vi "Send_Demand_controlword.vi"(0 "UDP connection ID out":refnum<k16>, 1 "Inner TRACK":T1={"Position"=100.0, "Rate"=100.0, "Acceleration"=100.0}, 2 "Middle TRACK":T1={"Position"=100.0, "Rate"=100.0, "Acceleration"=100.0}, 3 "Outer TRACK":T1={"Position"=100.0, "Rate"=100.0, "Acceleration"=100.0}, 5 "IP address in":u32=44, 12 "error in":errorcluster, 13 "ReadOnly":bool) -> (4 "UDP connection ID out":refnum<k16>, 6 "IP address out":u32=44, 8 "concatenated string":string, 14 "error out":errorcluster)   [LabVIEW 2017]
panel:
  in  "Inner P":cluster{dbl}
  in  "Middle P":cluster{dbl}
  in  "Outer P":cluster{dbl}
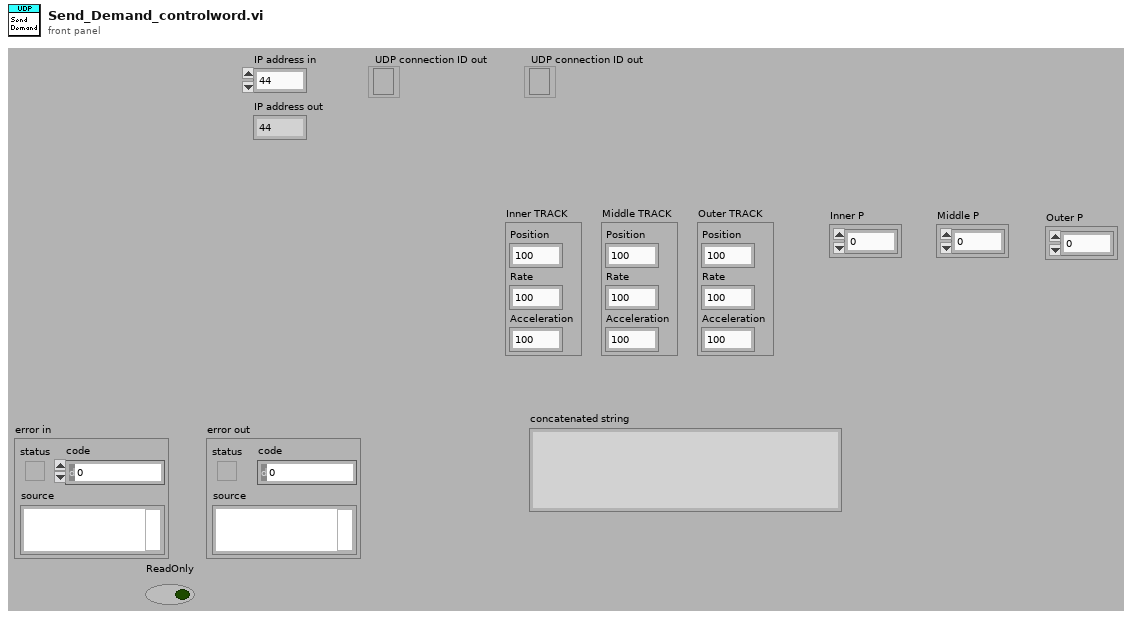
[diagram p1: front panel]
types:
  T1 = cluster{"Position":dbl, "Rate":dbl, "Acceleration":dbl}
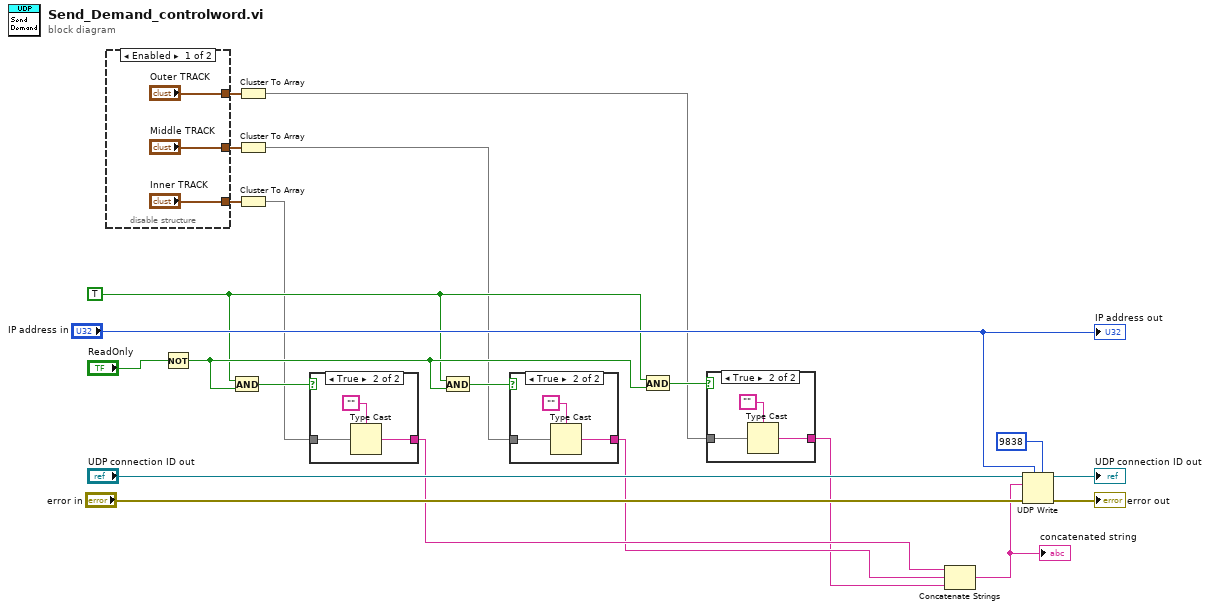
[diagram p0: block diagram]
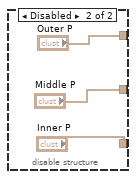
[diagram p2: hidden frame]
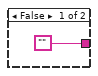
[diagram p3: hidden frame]
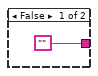
[diagram p4: hidden frame]
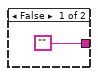
[diagram p5: hidden frame]
diagram:
  w5 = TRUE ("Axis3")
  n1 = disable-structure shown="Enabled" {
    disable-tunnel: ["Inner TRACK" "Inner P"] -> w8
    disable-tunnel: ["Middle TRACK" "Middle P"] -> w7
    disable-tunnel: ["Outer TRACK" "Outer P"] -> w6
    frame Enabled {
    }
    frame Disabled {
    }
  }
  n2 = Not(x="ReadOnly") -> (.not. x?=w12:bool)
  n3 = And(x=w5, y=w12) -> (x .and. y?=w15:bool)
  n4 = Cluster To Array(cluster=w6) -> (array=w2:dbl[])
  n5 = Cluster To Array(cluster=w7) -> (array=w3:dbl[])
  n6 = Cluster To Array(cluster=w8) -> (array=w4:dbl[])
  n7 = case shown="True" w15 {
    tunnel: w4 -> [_ w32]
    tunnel: ["" w30] -> w11
    frame False {
    }
    frame True {
      n8 = Type Cast(type="", x=w32) -> (*(type *) &x=w30:string)
    }
  }
  n9 = And(x=w5, y=w12) -> (x .and. y?=w14:bool)
  n10 = case shown="True" w14 {
    tunnel: w3 -> [_ w36]
    tunnel: ["" w34] -> w10
    frame False {
    }
    frame True {
      n11 = Type Cast(type="", x=w36) -> (*(type *) &x=w34:string)
    }
  }
  n12 = And(x=w5, y=w12) -> (x .and. y?=w13:bool)
  n13 = case shown="True" w13 {
    tunnel: w2 -> [_ w40]
    tunnel: ["" w38] -> w9
    frame False {
    }
    frame True {
      n14 = Type Cast(type="", x=w40) -> (*(type *) &x=w38:string)
    }
  }
  n15 = Concatenate Strings(w11, w10, w9) -> (w20:string)
  "concatenated string" <- w20
  n16 = UDP Write(address="IP address in", port or service name=u16 9838, connection ID="UDP connection ID out", data in=w20, 8:"error in") -> (error out=→"error out":errorcluster, 3:→"UDP connection ID out":refnum<k16>)  [unwired: 1 in]
  "IP address out" <- "IP address in"
